vi "ParsePololuTicStatus.vi"(11 "BytesIn":string) -> (3 "String":string)   [LabVIEW 2021]
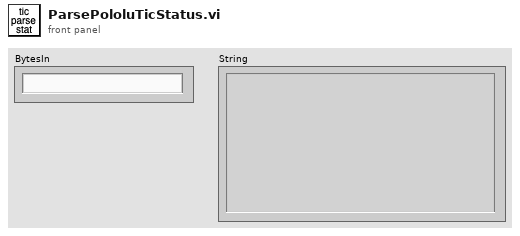
[diagram p1: front panel]
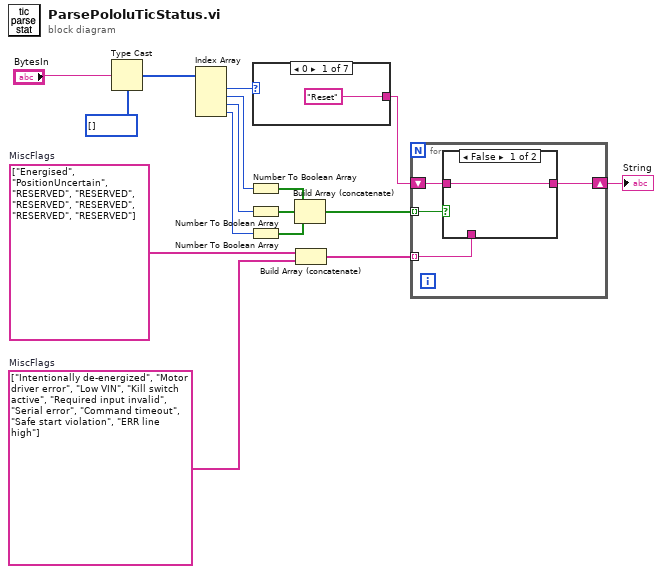
[diagram p0: block diagram]
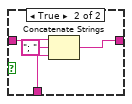
[diagram p2: hidden frame]
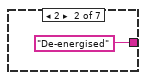
[diagram p3: hidden frame]
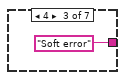
[diagram p4: hidden frame]
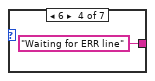
[diagram p5: hidden frame]
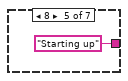
[diagram p6: hidden frame]
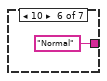
[diagram p7: hidden frame]
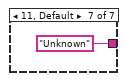
[diagram p8: hidden frame]
diagram:
  w14 = string[] ["Intentionally de-energized", "Motor driver error", "Low VIN", "Kill switch active", "Required input invalid", "Serial error", "Command timeout", "Safe start violation", "ERR line high"]  # MiscFlags
  w15 = string[] ["Energised", "PositionUncertain", "RESERVED", "RESERVED", "RESERVED", "RESERVED", "RESERVED", "RESERVED"]  # MiscFlags
  n1 = Type Cast(type=u8[] [], x="BytesIn") -> (*(type *) &x=w1:u8[])
  n2 = Index Array(array=w1) -> (element #1=w6:u8, element #2=w5:u8, element #3=w4:u8, element #4=w3:u8)  [unwired: 4 in]
  n3 = Number To Boolean Array(number=w5) -> (Boolean array=w13:bool[])
  n4 = Number To Boolean Array(number=w4) -> (Boolean array=w12:bool[])
  n5 = Number To Boolean Array(number=w3) -> (Boolean array=w11:bool[])
  n6 = case shown="0" w6 {
    tunnel: ["Reset" "De-energised" "Soft error" "Waiting for ERR line" "Starting up" "Normal" "Unknown"] -> w10
    frame 0 {
    }
    frame 2 {
    }
    frame 4 {
    }
    frame 6 {
    }
    frame 8 {
    }
    frame 10 {
    }
    frame 11, Default {
    }
  }
  n7 = Build Array (concatenate)(w13, w12, w11) -> (w9:bool[])
  n8 = Build Array (concatenate)(w15, w14) -> (w8:string[])
  n9 = for {
    shift-right: [w24] -> w7
    shift-left: w10 -> [w25]
    tunnel: w9 -> [w27] mode=indexing
    tunnel: w8 -> [w26] mode=indexing
    n10 = case shown="False" w27 {
      tunnel: w26 -> [_ w32]
      tunnel: w25 -> [w28 w31]
      tunnel: [w28 w29] -> w24
      frame False {
      }
      frame True {
        n11 = Concatenate Strings(w31, "; " ("string"), w32) -> (w29:string)
      }
    }
  }
  "String" <- w7
